vi "Graph.vi"(6 "Ring size (points) (1024)":u32=1024, 8 "error in (no error)":errorcluster, 9 "Store Ring? (f)":bool, 10 "Store History? (f)":bool, 11 "Readable in":refnum<class "Readable.lvclass">) -> (0 "error out":errorcluster, 1 "Ring Buffers":T5, 2 "History Buffers":T5, 3 "Readable out":refnum<class "Readable.lvclass">, 5 "Data Points":T1)   [LabVIEW 2023, in "Readable.lvclass"]
doc: "(Dynamic) Take a data point, then append it to an internal history buffer. Return the history buffer as a waveform array configured for graphing."
uses:
  Readable.lvclass
  TX Graph.ctl
  Data Points.ctl
  Data Point.ctl
  Time.ctl
  X.ctl
  Readable.lvclass/Readable.ctl
panel:
  # "Generate a waveform array for graphing."
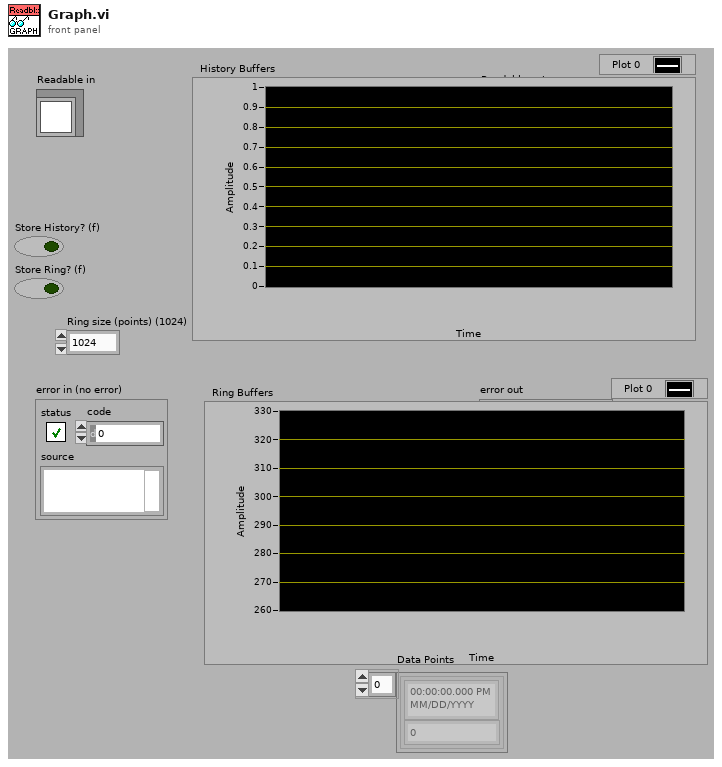
[diagram p1: front panel]
types:
  T1 = typedef "Readable.lvclass/Data Points.ctl" = T2[]
  T2 = typedef "Readable.lvclass/Data Point.ctl" = cluster{"t":T3, "x":T4}
  T3 = typedef "Readable.lvclass/Time.ctl" = timestamp
  T4 = typedef "Readable.lvclass/X.ctl" = dbl
  T5 = typedef "Readable.lvclass/TX Graph.ctl" = cluster{"Data Points":cluster{"t":timestamp, "x":dbl}[]}[]
  T6 = typedef "Readable.lvclass/Data Channels.ctl" = T7[]
  T7 = typedef "Readable.lvclass/Data Channel.ctl" = cluster{"Name":string, "Data Point":T2, "Unit":string}
  T8 = typedef "Readable.lvclass/Channel Names.ctl" = string[]
  T9 = cluster{"Data Points":cluster{"t":timestamp, "x":dbl}[]}
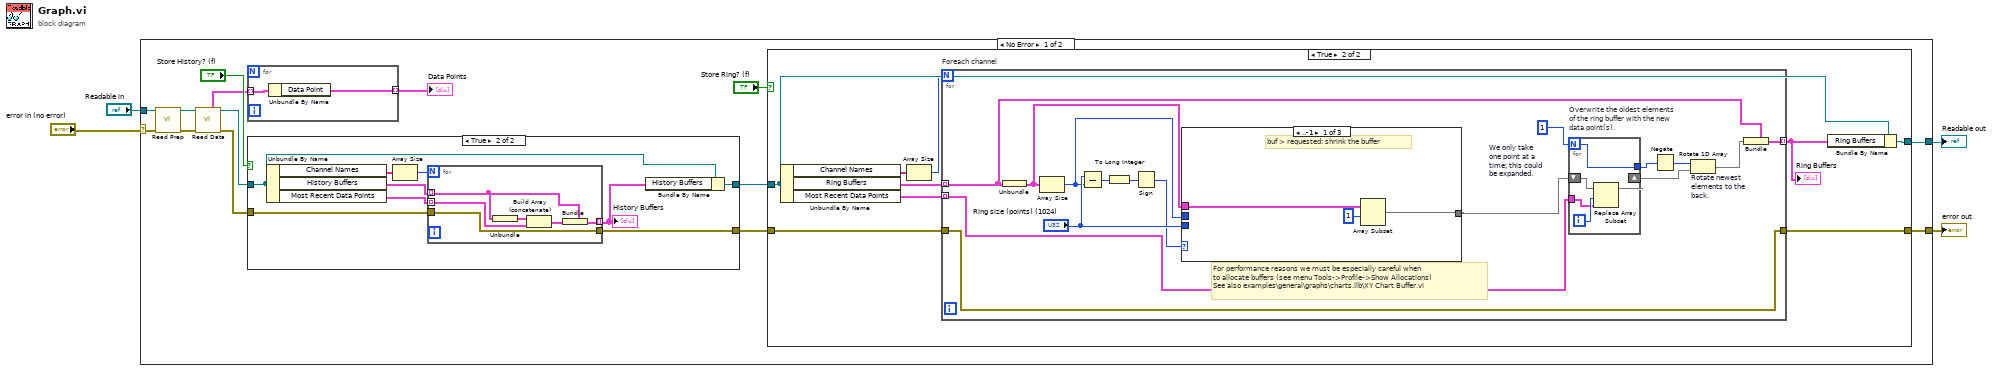
[diagram p0: block diagram]
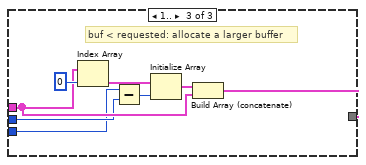
[diagram p4: hidden frame]
diagram:
  n1 = case shown="No Error" "error in (no error)" {
    selector: "error in (no error)" -> [w8 w83]
    tunnel: [w13 w83] -> w3
    tunnel: [w15 w82] -> w1
    tunnel: "Readable in" -> [w5 w82]
    frame No Error {
      n2 = call-dynamic "Read Prep.vi"("error in (no error)"=w8, "Readable in"=w5) -> ("error out"=w7:errorcluster, "Readable out"=w6:refnum<class "Readable.lvclass">)  [unwired: 8 in]
      n3 = call "Read Data.vi"("error in (no error)"=w7, "Readable in"=w6) -> ("error out"=w11:errorcluster, "Readable out"=w12:refnum<class "Readable.lvclass">, "Data Channels"=w10:T6)  [unwired: 3 in, 4 out]
      n4 = for {
        tunnel: w10 -> [w20] mode=indexing
        tunnel: [w19] -> w9 mode=indexing
        n5 = Unbundle By Name(w20) -> ("Data Point"=w19:T2)
      }
      "Data Points" <- w9
      n6 = case shown="True" "Store History? (f)" {
        tunnel: [w66 w75] -> w16
        tunnel: [w65 w74] -> w14
        tunnel: w11 -> [w65 w71]
        tunnel: w12 -> [w66 w69]
        frame False {
        }
        frame True {
          n7 = Unbundle By Name(w69) -> ("Channel Names"=w68:T8, "History Buffers"=w73:T5, "Most Recent Data Points"=w70:T1)
          n8 = Array Size(array=w68) -> (size(s)=w67:i32)
          n9 = for {
            N: w67 -> [_]
            tunnel: w71 -> [w81]
            tunnel: [w81] -> w74
            tunnel: [w79] -> w72 mode=indexing
            tunnel: w73 -> [w78] mode=indexing
            tunnel: w70 -> [w76] mode=indexing
            n10 = Unbundle(w78) -> ("Data Points"=w77:cluster{"t":timestamp, "x":dbl}[])
            n11 = Build Array (concatenate)(w77, w76) -> (w80:T2[])
            n12 = Bundle(cluster=w78, "Data Points"=w80) -> (w79:T9)
          }
          "History Buffers" <- w72
          n13 = Bundle By Name(cluster=w69, "History Buffers"=w72) -> (w75:refnum<class "Readable.lvclass">)
        }
      }
      n14 = case shown="True" "Store Ring? (f)" {
        tunnel: [w22 w31] -> w15
        tunnel: [w21 w30] -> w13
        tunnel: w14 -> [w21 w28]
        tunnel: w16 -> [w22 w26]
        frame False {
        }
        frame True {
          n15 = Unbundle By Name(w26) -> ("Channel Names"=w23:T8, "Ring Buffers"=w24:T5, "Most Recent Data Points"=w27:T1)
          n16 = Array Size(array=w23) -> (size(s)=w25:i32)
          n17 = for "Foreach channel" {
            N: w25 -> [_]
            tunnel: w28 -> [w47]
            tunnel: [w47] -> w30
            tunnel: [w46] -> w29 mode=indexing
            tunnel: w24 -> [w45] mode=indexing
            tunnel: w27 -> [w38] mode=indexing
            w37 = 1  # We only take one point at a time; this could be expanded.
            # "For performance reasons we must be especially careful when\nto allocate buffers (see menu Tools->Profile->Show Allocations)\nSee also examples\\general\\graphs\\charts.llb\\XY Chart Buffer.vi"
            n18 = Unbundle(w45) -> ("Data Points"=w44:cluster{"t":timestamp, "x":dbl}[])
            n19 = Array Size(array=w44) -> (size(s)=w41:i32)
            n20 = Subtract(x="Ring size (points) (1024)", y=w41) -> (x-y=w43:u32)
            n21 = To Long Integer(number=w43) -> (32bit integer=w40:i32)
            n22 = Sign(1:w40) -> (0:w39:i32)
            n23 = case shown="..-1" w39 {
              tunnel: [w54 w56 w60] -> w33
              tunnel: w44 -> [w55 w56 w61]
              tunnel: "Ring size (points) (1024)" -> [_ _ w58]
              tunnel: w41 -> [_ _ w59]
              frame ..-1 {
                # "buf > requested: shrink the buffer"
                n24 = Array Subset(array=w55, index=1) -> (w54:cluster{"t":timestamp, "x":dbl}[])  [unwired: 1 in]
              }
              frame 0 {
                # "buf == requested"
              }
              frame 1.. {
                # "buf < requested: allocate a larger buffer"
                n25 = Index Array(array=w61, index=0) -> (element=w63:cluster{"t":timestamp, "x":dbl})
                n26 = Subtract(x=w58, y=w59) -> (x-y=w57:u32)
                n27 = Initialize Array(w63, w57) -> (w62:cluster{"t":timestamp, "x":dbl}[])
                n28 = Build Array (concatenate)(w62, w61) -> (w60:cluster{"t":timestamp, "x":dbl}[])
              }
            }
            n29 = for "Overwrite the oldest elements\nof the ring buffer with the new\ndata point(s)." {
              N: w37 -> [w52]
              shift-right: [w48] -> w34
              shift-left: w33 -> [w49]
              tunnel: w38 -> [w50]
              tunnel: [w52] -> w36
              i -> [w51]
              n30 = Replace Array Subset(array=w49, new element=w50, index=w51) -> (w48:cluster{"t":timestamp, "x":dbl}[])
            }
            n31 = Negate(x=w36) -> (-x=w35:i32)
            n32 = Rotate 1D Array "Rotate newest \nelements to the \nback."(1:w34, 2:w35) -> (0:w32:cluster{"t":timestamp, "x":dbl}[])
            n33 = Bundle(cluster=w45, "Data Points"=w32) -> (w46:T9)
          }
          "Ring Buffers" <- w29
          n34 = Bundle By Name(cluster=w26, "Ring Buffers"=w29) -> (w31:refnum<class "Readable.lvclass">)
        }
      }
    }
    frame Error {
    }
  }
  "error out" <- w3
  "Readable out" <- w1
